vi "SENS_MULT_TSET_OUTP_DATA_S.vi"(0 "VISA IN":refnum<visa-resource-name>, 1 "ID":i32, 2 "Control Line Value":i32, 5 "error in":errorcluster, 7 "Channel":i32) -> (14 "VISA Out":refnum<visa-resource-name>, 19 "error out":errorcluster)   [LabVIEW 2018, in "PNA-X.lvlib"]
doc: "SENSe<cnum>:MULTiplexer<id>:TSET9:OUTPut[:DATA] <data> Superseded \nNote: This command is replaced with SENS:MULT:OUTP \n(Read-Write) Sets the control lines of the specified E5091A. Control lines, provided through a \nE5091A front panel connector, are used to control external equipment such as a part handler. See your \nE5091A documentation to learn more about control lines. \nParameters \n<cnum> Channel number of the measurement. If unspecified, value is set to 1. \n<id> Id of the E5091A test set. Choose from 1 or 2. Learn how to set ID value. \n<data> Data value used to set control lines. Values are obtained by adding weights \nfrom the following table that correspond to individual lines. HIGH =1; \nLOW=0. \n1785\n\nLine Weight \n1 1 \n2 2 \n3 4 \n4 8 \n5 16 \n6 32 \n7 64 \n8 128 \n0 - Sets all lines low \n255 - Sets all lines high \nExamples 'The following sets line 3 and 4 high. All other lines low. \nSENS:MULT1:TSET9:OUTP 12 \nQuery Syntax SENSe<cnum>:MULTiplexer<id>:TSET9:OUTPut[:DATA]? \nReturn Type Numeric \nDefault 0"
uses:
  PNA-X.lvlib
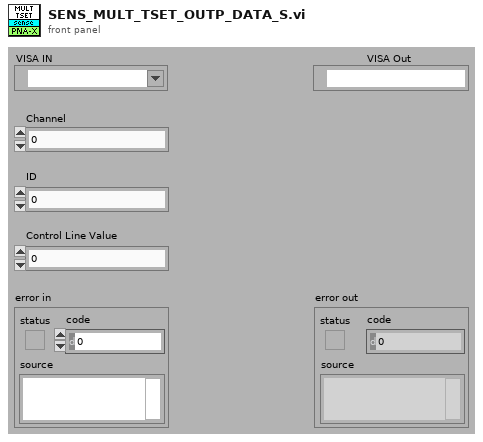
[diagram p1: front panel]
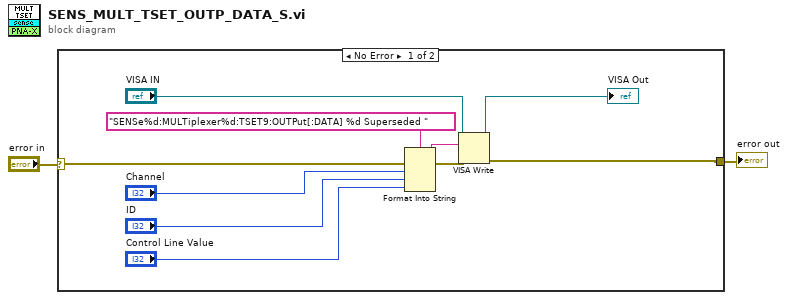
[diagram p0: block diagram]
diagram:
  n1 = case shown="No Error" "error in" {
    selector: "error in" -> [w12 w13]
    tunnel: [w7 w13] -> w1
    frame No Error {
      n2 = Format Into String(format string="SENSe%d:MULTiplexer%d:TSET9:OUTPut[:DATA] %d Superseded " ("Cmdline"), error in=w12, "Channel", "ID", "Control Line Value") -> (resulting string=w10:string, error out=w11:errorcluster)  [unwired: 1 in]
      n3 = VISA Write(VISA resource name="VISA IN", write buffer=w10, error in (no error)=w11) -> (VISA resource name out=→"VISA Out":refnum<visa-resource-name>, error out=w7:errorcluster)  [unwired: 1 out]
    }
    frame Error {
    }
  }
  "error out" <- w1
